vi "Graph.vi"(8 "error in (no error)":errorcluster, 10 "notifier out":refnum<notifier>, 11 "State in":T1={"State"=enum."Idle", "Start Time"=timestamp(0 s since 1904-01-01), "Configuration"={"Cycle Period"=0.0, "Manual Entry"=0.0, "Output Device"=enum."Default", "EPOS4 Settings"={"VISA resource name"="", "axis"={"keyHandle"=1, "nodeId"=1}, "Simulated?"=FALSE}}, "Current Time"=timestamp(0 s since 1904-01-01), "First Iteration"=FALSE, "Data"={"Centrifuge Speed"=0.0}, "Process Name"="", "Centrifuge On?"=enum."Off", "Output Error"=FALSE, "Log Started"=FALSE}) -> (0 "error out":errorcluster, 3 "State out":T1={"State"=enum."Idle", "Start Time"=timestamp(0 s since 1904-01-01), "Configuration"={"Cycle Period"=0.0, "Manual Entry"=0.0, "Output Device"=enum."Default", "EPOS4 Settings"={"VISA resource name"="", "axis"={"keyHandle"=1, "nodeId"=1}, "Simulated?"=FALSE}}, "Current Time"=timestamp(0 s since 1904-01-01), "First Iteration"=FALSE, "Data"={"Centrifuge Speed"=0.0}, "Process Name"="", "Centrifuge On?"=enum."Off", "Output Error"=FALSE, "Log Started"=FALSE})   [LabVIEW 2018, in "Centrifuge Module.lvlib" / "Centrifuge Module Engine.lvlib"]
uses:
  Centrifuge Module Engine.lvlib
  State Cluster.ctl
  State Enum.ctl
  Centrifuge Module Settings Cluster.ctl
  EPOS4/Controls/Device Selection.ctl
  EPOS4/Controls/EPOS Communication Settings.ctl
  Centrifuge Module.lvlib
  EPOS4/EPOS4.lvlib
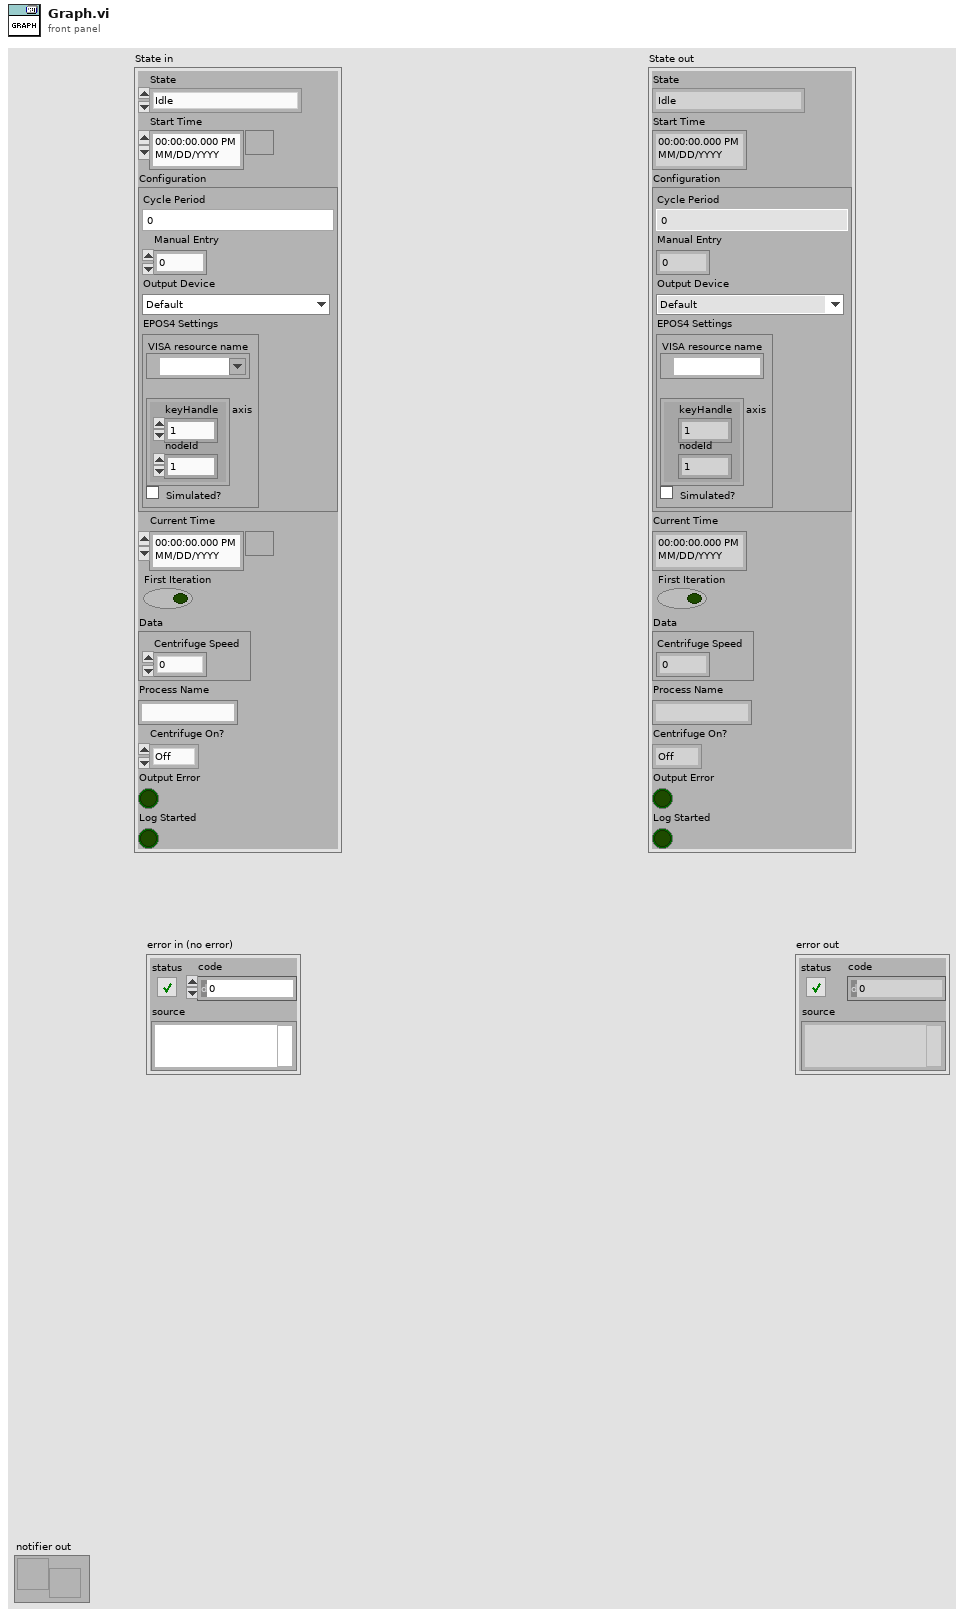
[diagram p1: front panel]
types:
  T1 = typedef "Centrifuge Module.lvlib/Centrifuge Module Engine.lvlib/State Cluster.ctl" = cluster{"State":T2, "Start Time":timestamp, "Configuration":T3, "Current Time":timestamp, "First Iteration":bool, "Data":cluster{"Centrifuge Speed":dbl}, "Process Name":string, "Centrifuge On?":enum16{"Off", "On", "Not Initialized"}, "Output Error":bool, "Log Started":bool}
  T2 = typedef "Centrifuge Module.lvlib/Centrifuge Module Engine.lvlib/State Enum.ctl" = enum16{"Measuring", "Idle", "Paused"}
  T3 = typedef "Centrifuge Module.lvlib/Centrifuge Module Settings Cluster.ctl" = cluster{"Cycle Period":dbl, "Manual Entry":dbl, "Output Device":T4, "EPOS4 Settings":T5}
  T4 = typedef "Device Selection.ctl" = enum16{"Default", "EPOS4"}
  T5 = typedef "EPOS4.lvlib/EPOS Communication Settings.ctl" = cluster{"VISA resource name":refnum<visa-resource-name>, "axis":cluster{"keyHandle":u32, "nodeId":u16}, "Simulated?":bool}
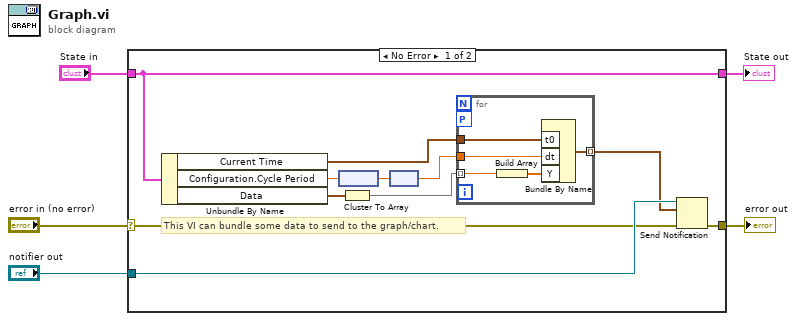
[diagram p0: block diagram]
diagram:
  n1 = case shown="No Error" "error in (no error)" {
    selector: "error in (no error)" -> [w13 w23]
    tunnel: [w12 w23] -> w4
    tunnel: "State in" -> [w16 w22]
    tunnel: [w16 w22] -> w2
    tunnel: "notifier out" -> [w14 _]
    frame No Error {
      # "This VI can bundle some data to send to the graph/chart."
      n2 = Unbundle By Name(w16) -> ("Current Time"=w11:timestamp, "Configuration.Cycle Period"=w10:dbl, "Data"=w15:cluster{"Centrifuge Speed":dbl})
      n3 = node(w10) -> (w9:dbl[unit])
      n4 = Cluster To Array(cluster=w15) -> (array=w7:dbl[])
      n5 = node(w9) -> (w8:dbl)
      n6 = for {
        tunnel: w11 -> [w21]
        tunnel: w8 -> [w20]
        tunnel: w7 -> [w19] mode=indexing
        tunnel: [w17] -> w6 mode=indexing
        workers-P: _ -> [_]
        n7 = Build Array(w19) -> (w18:dbl[])
        n8 = Bundle By Name("t0"=w21, "dt"=w20, "Y"=w18) -> (w17:waveform(dbl))  [unwired: 1 in]
      }
      n9 = Send Notification(notification=w6, notifier=w14, error in (no error)=w13) -> (error out=w12:errorcluster)  [unwired: 1 out]
    }
    frame Error {
    }
  }
  "error out" <- w4
  "State out" <- w2
